vi "Load.vi"(0 "Robot Event Local Log in":refnum<class "Robot Event SystemLink.lvclass">, 1 "Event Parameters":T1[](array[typedef]), 5 "error in (no error)":errorcluster) -> (14 "Robot Event Local Log out":refnum<class "Robot Event SystemLink.lvclass">, 19 "error out":errorcluster)   [LabVIEW 2019, in "Robot Event SystemLink.lvclass"]
uses:
  Robot Event SystemLink.lvclass
  Robot Event/Event Parameters.ctl
  Robot Event SystemLink.lvclass/Robot Event SystemLink.ctl
  Robot Event/Robot Event.lvclass
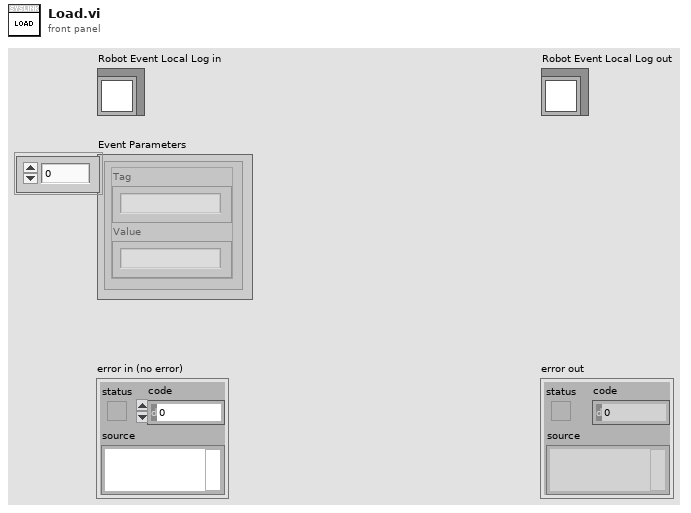
[diagram p1: front panel]
types:
  T1 = typedef "Robot Event.lvclass/Event Parameters.ctl" = cluster{"Tag":string, "Value":string}
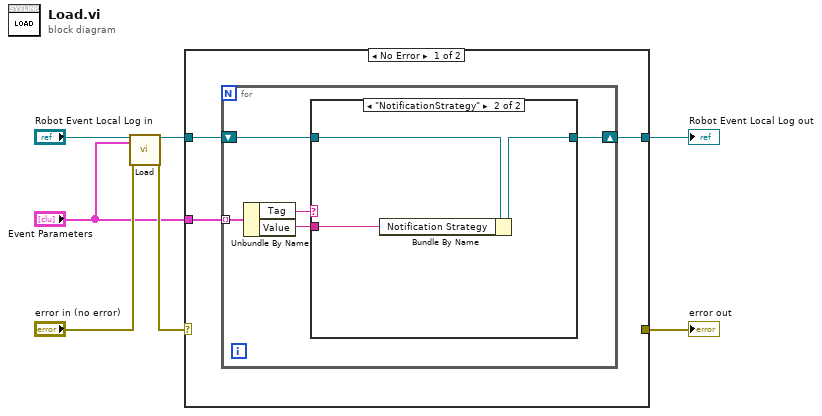
[diagram p0: block diagram]
diagram:
  n1 = call-parent "Load.vi"("Robot Event in"="Robot Event Local Log in", "Event Parameters"="Event Parameters", "error in (no error)"="error in (no error)") -> ("Robot Event out"=w4:refnum<class "Robot Event SystemLink.lvclass">, "error out"=w3:errorcluster)  [unwired: 15 in]
  n2 = case shown="No Error" w3 {
    selector: w3 -> [_ w21]
    tunnel: [_ w21] -> w7
    tunnel: [w9 w20] -> w6
    tunnel: w4 -> [w10 w20]
    tunnel: "Event Parameters" -> [w8 _]
    frame No Error {
      n3 = for {
        shift-right: [w14] -> w9
        shift-left: w10 -> [w15]
        tunnel: w8 -> [w13] mode=indexing
        n4 = Unbundle By Name(w13) -> ("Tag"=w12:string, "Value"=w11:string)
        n5 = case shown="\"NotificationStrategy\"" w12 {
          tunnel: w15 -> [w16 w19]
          tunnel: [w16 w18] -> w14
          tunnel: w11 -> [_ w17]
          frame Default {
          }
          frame "NotificationStrategy" {
            n6 = Bundle By Name(cluster=w19, "Notification Strategy"=w17) -> (w18:refnum<class "Robot Event SystemLink.lvclass">)
          }
        }
      }
    }
    frame Error {
    }
  }
  "error out" <- w7
  "Robot Event Local Log out" <- w6
